vi "Fill To.vi"(5 "Col":i32, 6 "Attributes":T1, 8 "error in (no error)":errorcluster, 10 "Char":string, 11 "TermLine in":refnum<class "TermLine.lvclass">) -> (0 "error out":errorcluster, 3 "TermLine out":refnum<class "TermLine.lvclass">)   [LabVIEW 2020, in "Terminal.lvlib" / "TermLine.lvclass"]
uses:
  TermLine.lvclass
  TermLine.lvclass/TermLine.ctl
  Term Char.ctl
  Terminal.lvlib
  Text Attributes.ctl
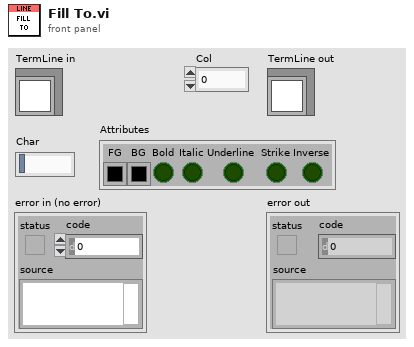
[diagram p1: front panel]
types:
  T1 = typedef "Terminal.lvlib/Text Attributes.ctl" = cluster{"FG":u32, "BG":u32, "Bold":bool, "Italic":bool, "Underline":bool, "Strike":bool, "Inverse":bool}
  T2 = typedef "Terminal.lvlib/Term Char.ctl" = cluster{"Char":string, "Attributes":T1}
  T3 = typedef "Terminal.lvlib/TermLine.lvclass/Ref Data.ctl" = cluster{"Chars":T2[], "Width":i32}
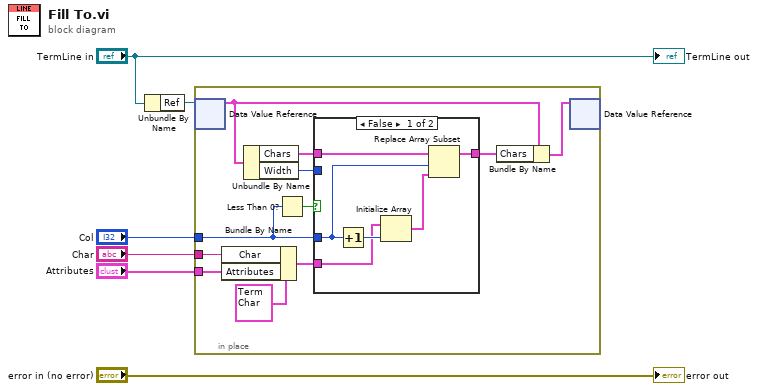
[diagram p0: block diagram]
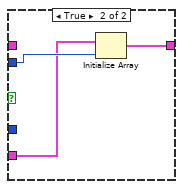
[diagram p2: hidden frame]
diagram:
  n1 = Unbundle By Name("TermLine in") -> ("Ref"=w5:refnum<data-value>)
  n2 = in-place {
    in-place-border: "Col" -> [w11]
    in-place-border: "Char" -> [w9]
    in-place-border: "Attributes" -> [w8]
    n3 = in-place-dvr #1(w5) -> (w17:T3)  [unwired: 1 out]
    n4 = Bundle By Name(cluster=T2 {"Char"=" ", "Attributes"={"FG"=16777216, "BG"=16777216, "Bold"=FALSE, "Italic"=FALSE, "Underline"=FALSE, "Strike"=FALSE, "Inverse"=FALSE}} ("Term Char"), "Char"=w9, "Attributes"=w8) -> (w7:T2)
    n5 = Unbundle By Name(w17) -> ("Chars"=w15:T2[], "Width"=w13:i32)
    n6 = Less Than 0?(x=w11) -> (x < 0?=w14:bool)
    n7 = case shown="False" w14 {
      tunnel: w15 -> [w23 _]
      tunnel: w13 -> [_ w26]
      tunnel: [w18 w25] -> w12
      tunnel: w11 -> [w19 _]
      tunnel: w7 -> [w21 w24]
      frame False {
        n8 = Increment(x=w19) -> (x+1=w22:i32)
        n9 = Initialize Array(w21, w22) -> (w20:T2[])
        n10 = Replace Array Subset(array=w23, new element=w20, index=w19) -> (w18:T2[])
      }
      frame True {
        n11 = Initialize Array(w24, w26) -> (w25:T2[])
      }
    }
    n12 = Bundle By Name(cluster=w17, "Chars"=w12) -> (w16:T3)
    n13 = in-place-dvr #1(w16) -> ()  [unwired: 2 out]
  }
  "error out" <- "error in (no error)"
  "TermLine out" <- "TermLine in"
